vi "Write Controller Options.vi"(7 "Unit ID (A)":string="A", 8 "error in":errorcluster, 9 "Software Version":u8, 10 "Read/Write Options":T1 {"Controller Select" items=["No controller"=0, "Volumetric Flow"=36, "Mass Flow"=37, "Absolute Pressure"=34, "Gauge Pressure"=38, "Differential Pressure"=39]}, 11 "VISA Session In":refnum<visa-resource-name>="Alicat") -> (0 "error out":errorcluster, 3 "VISA Session Out":refnum<visa-resource-name>)   [LabVIEW 2015]
doc: "Writes the controller options to a connected Alicat:Selected control variable, setpoint source, and auto tare on/off."
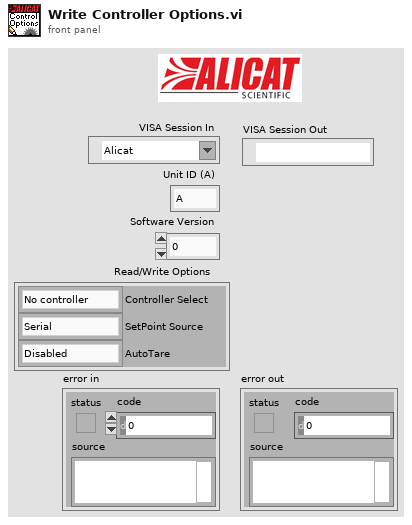
[diagram p1: front panel]
types:
  T1 = cluster{"Controller Select":u16, "SetPoint Source":enum8{"Serial", "Local", "Analog", "Unknown"}, "AutoTare":enum16{"Disabled", "Enabled"}}
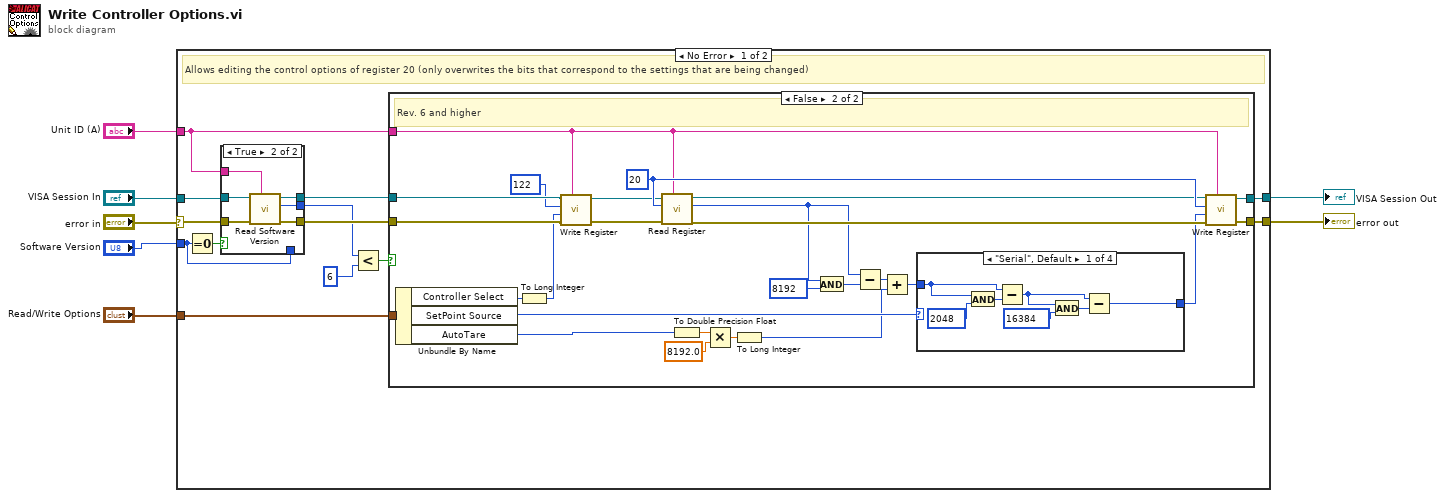
[diagram p0: block diagram]
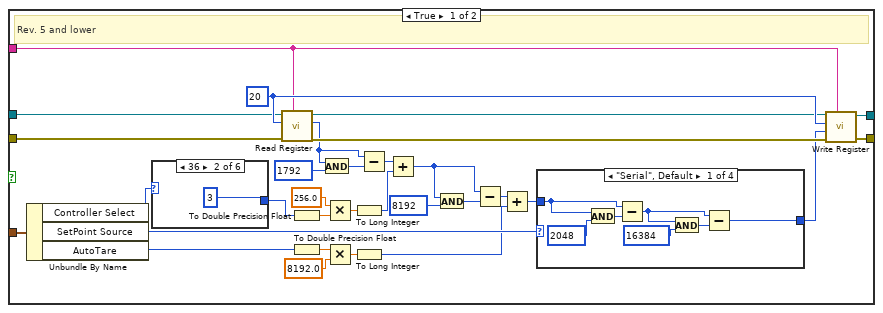
[diagram p2: hidden frame]
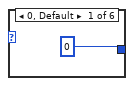
[diagram p3: hidden frame]
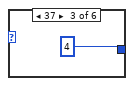
[diagram p4: hidden frame]
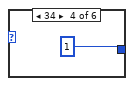
[diagram p5: hidden frame]
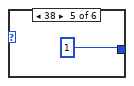
[diagram p6: hidden frame]
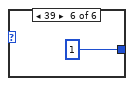
[diagram p7: hidden frame]
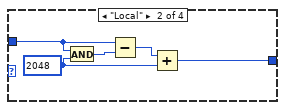
[diagram p8: hidden frame]
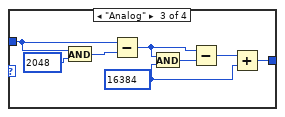
[diagram p9: hidden frame]
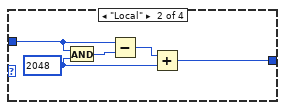
[diagram p11: hidden frame]
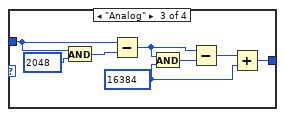
[diagram p12: hidden frame]
diagram:
  n1 = case shown="No Error" "error in" {
    selector: "error in" -> [w14 w135]
    tunnel: [w20 w136] -> w7
    tunnel: [w19 w135] -> w6
    tunnel: "VISA Session In" -> [w13 w136]
    tunnel: "Unit ID (A)" -> [w8 _]
    tunnel: "Read/Write Options" -> [w18 _]
    tunnel: "Software Version" -> [w12 _]
    frame No Error {
      # "Allows editing the control options of register 20 (only overwrites the bits that correspond to the settings that are being changed)"
      n2 = Equal To 0?(x=w12) -> (x = 0?=w17:bool)
      n3 = case shown="True" w17 {
        tunnel: w14 -> [w127 w134]
        tunnel: w13 -> [w126 w133]
        tunnel: w8 -> [_ w132]
        tunnel: [w127 w131] -> w15
        tunnel: [w126 w130] -> w16
        tunnel: [w128 w129] -> w9
        tunnel: w12 -> [w128 _]
        frame False {
        }
        frame True {
          n4 = call "Read Software Version.vi"("Unit ID (A)"=w132, "error in"=w134, "VISA Session In"=w133) -> ("error out"=w131:errorcluster, "Software Version"=w129:u8, "VISA Session Out"=w130:refnum<visa-resource-name>)  [unwired: 6 in]
        }
      }
      n5 = Less?(x=w9, y=u8 6) -> (x < y?=w10:bool)
      n6 = case shown="False" w10 {
        tunnel: [w48 w101] -> w20
        tunnel: [w47 w100] -> w19
        tunnel: w18 -> [w46 w99]
        tunnel: w16 -> [w25 w85]
        tunnel: w15 -> [w24 w84]
        tunnel: w8 -> [w21 w86]
        frame True {
          w51 = u16 20 ("register")
          # "Rev. 5 and lower"
          n7 = Unbundle By Name(w46) -> ("Controller Select"=w23:u16, "SetPoint Source"=w45:enum8{"Serial", "Local", "Analog", "Unknown"}, "AutoTare"=w34:enum16{"Disabled", "Enabled"})
          n8 = case shown="36" w23 {
            tunnel: [0 ("y") 3 ("y") 4 ("y") 1 ("y") 1 ("y") 1 ("y")] -> w22
            frame 0, Default {
            }
            frame 36 {
            }
            frame 37 {
            }
            frame 34 {
            }
            frame 38 {
            }
            frame 39 {
            }
          }
          n9 = call "Read Register.vi"("Unit ID (A)"=w21, "error in"=w24, "Register address"=w51, "VISA Session In"=w25) -> ("error out"=w50:errorcluster, "Register Value (I32)"=w39:i32, "VISA Session Out"=w49:refnum<visa-resource-name>)  [unwired: 5 in]
          n10 = To Double Precision Float(number=w22) -> (double precision float=w44:dbl)
          n11 = To Double Precision Float(number=w34) -> (double precision float=w35:dbl)
          n12 = And(x=w39, y=1792) -> (x .and. y?=w40:i32)
          n13 = Multiply(x=256.0, y=w44) -> (x*y=w42:dbl)
          n14 = Multiply(x=w35, y=8192.0 ("x")) -> (x*y=w33:dbl)
          n15 = To Long Integer(number=w42) -> (32bit integer=w37:i32)
          n16 = To Long Integer(number=w33) -> (32bit integer=w28:i32)
          n17 = Subtract(x=w39, y=w40) -> (x-y=w38:i32)
          n18 = Add(x=w38, y=w37) -> (x+y=w30:i32)
          n19 = And(x=w30, y=8192) -> (x .and. y?=w31:i32)
          n20 = Subtract(x=w30, y=w31) -> (x-y=w29:i32)
          n21 = Add(x=w29, y=w28) -> (x+y=w27:i32)
          n22 = case shown="\"Serial\", Default" w45 {
            tunnel: w27 -> [w59 w68 w75 w78]
            tunnel: [w58 w65 w70 w78] -> w26
            frame "Serial", Default {
              n23 = And(x=w59, y=2048) -> (x .and. y?=w63:i32)
              n24 = Subtract(x=w59, y=w63) -> (x-y=w61:i32)
              n25 = And(x=w61, y=16384) -> (x .and. y?=w62:i32)
              n26 = Subtract(x=w61, y=w62) -> (x-y=w58:i32)
            }
            frame "Local" {
              w66 = 2048 ("y")
              n27 = And(x=w68, y=w66) -> (x .and. y?=w69:i32)
              n28 = Subtract(x=w68, y=w69) -> (x-y=w67:i32)
              n29 = Add(x=w67, y=w66) -> (x+y=w65:i32)
            }
            frame "Analog" {
              w71 = 16384 ("y")
              n30 = And(x=w75, y=2048) -> (x .and. y?=w76:i32)
              n31 = Subtract(x=w75, y=w76) -> (x-y=w73:i32)
              n32 = And(x=w73, y=w71) -> (x .and. y?=w74:i32)
              n33 = Subtract(x=w73, y=w74) -> (x-y=w72:i32)
              n34 = Add(x=w72, y=w71) -> (x+y=w70:i32)
            }
            frame "Unknown" {
            }
          }
          n35 = call "Write Register.vi"("Unit ID (A)"=w21, "error in"=w50, "Register Value"=w26, "Register address"=w51, "VISA Session In"=w49) -> ("error out"=w47:errorcluster, "VISA Session Out"=w48:refnum<visa-resource-name>)  [unwired: 4 in, 1 out]
        }
        frame False {
          w104 = u16 20 ("register")
          # "Rev. 6 and higher"
          n36 = Unbundle By Name(w99) -> ("Controller Select"=w80:u16, "SetPoint Source"=w98:enum8{"Serial", "Local", "Analog", "Unknown"}, "AutoTare"=w95:enum16{"Disabled", "Enabled"})
          n37 = To Long Integer(number=w80) -> (32bit integer=w79:i32)
          n38 = call "Write Register.vi"("Unit ID (A)"=w86, "error in"=w84, "Register Value"=w79, "Register address"=u16 122, "VISA Session In"=w85) -> ("error out"=w82:errorcluster, "VISA Session Out"=w83:refnum<visa-resource-name>)  [unwired: 4 in, 1 out]
          n39 = call "Read Register.vi"("Unit ID (A)"=w86, "error in"=w82, "Register address"=w104, "VISA Session In"=w83) -> ("error out"=w103:errorcluster, "Register Value (I32)"=w87:i32, "VISA Session Out"=w102:refnum<visa-resource-name>)  [unwired: 5 in]
          n40 = To Double Precision Float(number=w95) -> (double precision float=w96:dbl)
          n41 = Multiply(x=w96, y=8192.0 ("x")) -> (x*y=w94:dbl)
          n42 = To Long Integer(number=w94) -> (32bit integer=w90:i32)
          n43 = And(x=w87, y=8192) -> (x .and. y?=w92:i32)
          n44 = Subtract(x=w87, y=w92) -> (x-y=w91:i32)
          n45 = Add(x=w91, y=w90) -> (x+y=w89:i32)
          n46 = case shown="\"Serial\", Default" w98 {
            tunnel: w89 -> [w106 w115 w122 w125]
            tunnel: [w105 w112 w117 w125] -> w88
            frame "Serial", Default {
              n47 = And(x=w106, y=2048) -> (x .and. y?=w110:i32)
              n48 = Subtract(x=w106, y=w110) -> (x-y=w108:i32)
              n49 = And(x=w108, y=16384) -> (x .and. y?=w109:i32)
              n50 = Subtract(x=w108, y=w109) -> (x-y=w105:i32)
            }
            frame "Local" {
              w113 = 2048 ("y")
              n51 = And(x=w115, y=w113) -> (x .and. y?=w116:i32)
              n52 = Subtract(x=w115, y=w116) -> (x-y=w114:i32)
              n53 = Add(x=w114, y=w113) -> (x+y=w112:i32)
            }
            frame "Analog" {
              w118 = 16384 ("y")
              n54 = And(x=w122, y=2048) -> (x .and. y?=w123:i32)
              n55 = Subtract(x=w122, y=w123) -> (x-y=w120:i32)
              n56 = And(x=w120, y=w118) -> (x .and. y?=w121:i32)
              n57 = Subtract(x=w120, y=w121) -> (x-y=w119:i32)
              n58 = Add(x=w119, y=w118) -> (x+y=w117:i32)
            }
            frame "Unknown" {
            }
          }
          n59 = call "Write Register.vi"("Unit ID (A)"=w86, "error in"=w103, "Register Value"=w88, "Register address"=w104, "VISA Session In"=w102) -> ("error out"=w100:errorcluster, "VISA Session Out"=w101:refnum<visa-resource-name>)  [unwired: 4 in, 1 out]
        }
      }
    }
    frame Error {
    }
  }
  "error out" <- w6
  "VISA Session Out" <- w7
